vi "Listen.vi"(7 "Listen Address (0=All)":u32 format="%08x", 8 "error in (no error)":errorcluster, 10 "Listen Port (80)":u16=80, 11 "API Queue":refnum<queue>) -> (0 "error out":errorcluster)   [LabVIEW 2023, in "Server.lvclass"]
doc: "Listen on the specified Port. (or on the port stored in the 'Listen Port' VIG)\nAccepts all incoming REST requests, handling them internally if possible. (e.g. static file, control reference endpoint, or event endpoint)\n\nListen Address defaults to all interfaces, either use 'String to IP' to get the network address or 0xCA000001 to only listen on localhost. (The Hex value for 127.0.0.1)"
uses:
  Server.lvclass
  API Message/API Message.lvclass
  Log/Log_Facilities.ctl
  Server.lvclass/Server.ctl
  Log/Log.lvclass
  Request/Request.lvclass
  Response/Response.lvclass
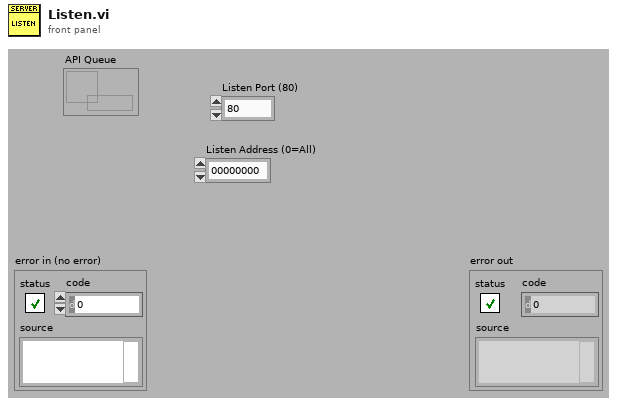
[diagram p1: front panel]
types:
  T1 = typedef "Log.lvclass/Log_Facilities.ctl" = string
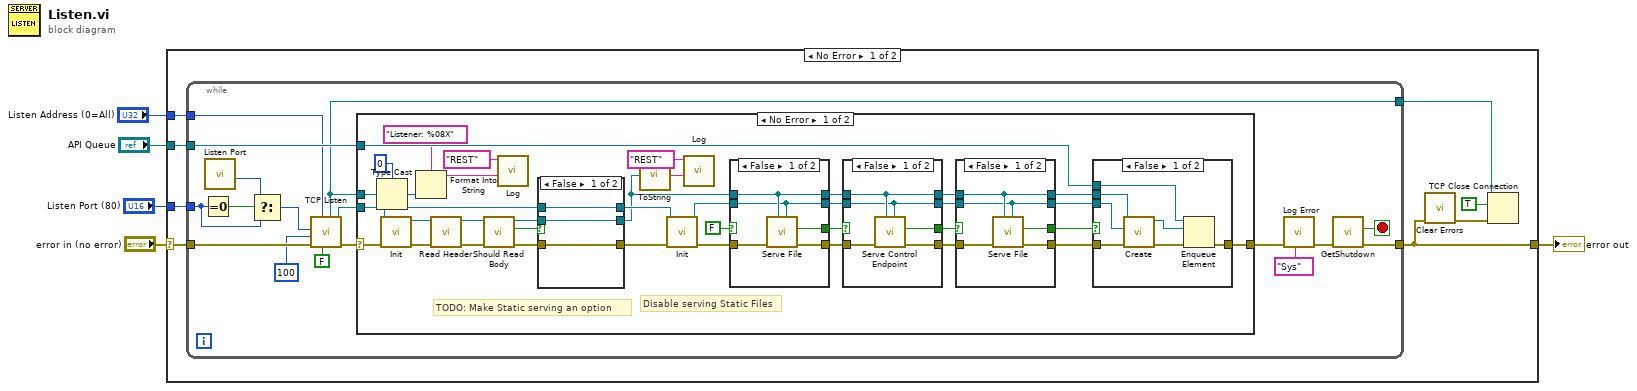
[diagram p0: block diagram]
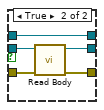
[diagram p6: hidden frame]
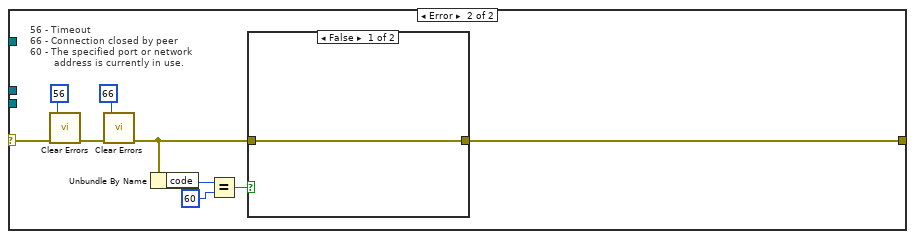
[diagram p7: hidden frame]
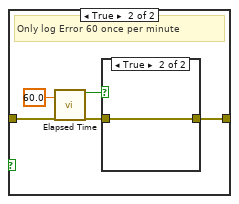
[diagram p8: hidden frame]
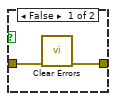
[diagram p9: hidden frame]
diagram:
  n1 = case shown="No Error" "error in (no error)" {
    selector: "error in (no error)" -> [w13 w129]
    tunnel: [w9 w129] -> w4
    tunnel: "API Queue" -> [w12 _]
    tunnel: "Listen Port (80)" -> [w7 _]
    tunnel: "Listen Address (0=All)" -> [w6 _]
    frame No Error {
      n2 = while {
        tunnel: w13 -> [w30]
        tunnel: [w21] -> w9
        tunnel: w12 -> [w23]
        tunnel: [w14] -> w11
        tunnel: w7 -> [w17]
        tunnel: w6 -> [w15]
        stop <- w20 stop-if-true
        n3 = Equal To 0?(x=w17) -> (x = 0?=w19:bool)
        n4 = call "Listen Port.vi"() -> ("Port out"=w18:u16)  [unwired: 11 in]
        n5 = Select(t=w18, s=w19, f=w17) -> (s? t:f=w16:u16)
        n6 = call <vilib>:"TCP Listen.vi"("resolve remote address (T)"=FALSE, "net address"=w15, "error in (no error)"=w30, "timeout ms (wait forever: -1)"=100 ("port"), "port"=w16) -> ("error out"=w27:errorcluster, "connection ID"=w25:refnum<k5>, "listener ID"=w14:refnum<k5>)  [unwired: 2 in, 2 out]
        n7 = case shown="No Error" w27 {
          selector: w27 -> [w67 w117]
          tunnel: w25 -> [w36 _]
          tunnel: [w54 w111] -> w26
          tunnel: w23 -> [w51 _]
          tunnel: w14 -> [w32 _]
          frame No Error {
            # "TODO: Make Static serving an option"
            # "Disable serving Static Files"
            n8 = Type Cast(type=u32 0, x=w32) -> (*(type *) &x=w34:u32)
            n9 = call "Init.vi"("error in (no error)"=w67, "Socket"=w36) -> ("error out"=w60:errorcluster, "Request out"=w62:refnum<class "Request.lvclass">)  [unwired: 8 in]
            n10 = Format Into String(format string="Listener: %08X", w34) -> (resulting string=w35:string)  [unwired: 2 in, 1 out]
            n11 = call "Read Header.vi"("error in (no error)"=w60, "Request in"=w62) -> ("error out"=w59:errorcluster, "Request out"=w61:refnum<class "Request.lvclass">)  [unwired: 8 in]
            n12 = call "Should Read Body.vi"("error in (no error)"=w59, "Request in"=w61) -> ("error out"=w66:errorcluster, "Read Body?"=w64:bool, "Request out"=w65:refnum<class "Request.lvclass">)  [unwired: 7 in]
            n13 = call "Log.vi"("Message"=w35, "Facility"=T1 "REST") -> ()  [unwired: 9 in, 1 out]
            n14 = case shown="False" w64 {
              tunnel: w66 -> [w104 w110]
              tunnel: [w104 w109] -> w58
              tunnel: w65 -> [w105 w108]
              tunnel: [w105 w107] -> w53
              tunnel: w36 -> [w103 w106]
              tunnel: [w103 w106] -> w63
              frame False {
              }
              frame True {
                n15 = call "Read Body.vi"("error in (no error)"=w110, "Request in"=w108) -> ("error out"=w109:errorcluster, "Request out"=w107:refnum<class "Request.lvclass">)  [unwired: 8 in]
              }
            }
            n16 = call "ToString.vi"("Request"=w53) -> ("String"=w57:string)
            n17 = call "Init.vi"("error in (no error)"=w58, "Socket"=w63) -> ("error out"=w56:errorcluster, "Response out"=w52:refnum<class "Response.lvclass">)  [unwired: 8 in]
            n18 = call "Log.vi"("Message"=w57, "Facility"=T1 "REST") -> ()  [unwired: 9 in, 1 out]
            n19 = case shown="False" FALSE {
              selector: FALSE -> [_ w101]
              tunnel: [w98 w102] -> w46
              tunnel: w53 -> [w95 w100]
              tunnel: w52 -> [w94 w99]
              tunnel: w56 -> [w97 w102]
              tunnel: [w96 w101] -> w47
              tunnel: [w95 w100] -> w49
              tunnel: [w94 w99] -> w48
              frame False {
                n20 = call "Serve File.vi"("Response"=w94, "Request"=w95, "error in (no error)"=w97) -> ("error out"=w98:errorcluster, "Handled?"=w96:bool)  [unwired: 7 in]
              }
              frame True {
              }
            }
            n21 = case shown="False" w47 {
              selector: w47 -> [_ w84]
              tunnel: [w80 w85] -> w41
              tunnel: w49 -> [w79 w83]
              tunnel: w48 -> [w78 w82]
              tunnel: w46 -> [w81 w85]
              tunnel: [w77 w84] -> w42
              tunnel: [w79 w83] -> w44
              tunnel: [w78 w82] -> w43
              frame False {
                n22 = call "Serve Control Endpoint.vi"("Response"=w78, "Request"=w79, "error in (no error)"=w81) -> ("error out"=w80:errorcluster, "Handled?"=w77:bool)  [unwired: 7 in]
              }
              frame True {
              }
            }
            n23 = case shown="False" w42 {
              selector: w42 -> [_ w75]
              tunnel: [w72 w76] -> w40
              tunnel: w44 -> [w69 w74]
              tunnel: w43 -> [w68 w73]
              tunnel: w41 -> [w71 w76]
              tunnel: [w70 w75] -> w45
              tunnel: [w69 w74] -> w38
              tunnel: [w68 w73] -> w39
              frame False {
                n24 = call "Serve File.vi"("Response"=w68, "Request"=w69, "error in (no error)"=w71) -> ("error out"=w72:errorcluster, "Handled?"=w70:bool)  [unwired: 7 in]
              }
              frame True {
              }
            }
            n25 = case shown="False" w45 {
              tunnel: [w88 w93] -> w54
              tunnel: w38 -> [w92 _]
              tunnel: w39 -> [w91 _]
              tunnel: w40 -> [w87 w93]
              tunnel: w51 -> [w90 _]
              frame False {
                n26 = call "Create.vi"("error in (no error)"=w87, "Response"=w91, "Request"=w92) -> ("error out"=w86:errorcluster, "API Message out"=w89:refnum<class "API Message.lvclass">)  [unwired: 7 in]
                n27 = Enqueue Element(queue=w90, element=w89, error in (no error)=w86) -> (error out=w88:errorcluster)  [unwired: 1 in, 2 out]
              }
              frame True {
              }
            }
          }
          frame Error {
            # "56 - Timeout\n66 - Connection closed by peer\n60 - The specified port or network \n        address is currently in use."
            n28 = call <vilib>:"Clear Errors.vi"("error in (no error)"=w117, "specific error code to clear (0: all)"=56) -> ("error out"=w116:errorcluster)  [unwired: 4 in, 1 out]
            n29 = call <vilib>:"Clear Errors.vi"("error in (no error)"=w116, "specific error code to clear (0: all)"=66) -> ("error out"=w112:errorcluster)  [unwired: 4 in, 1 out]
            n30 = Unbundle By Name(w112) -> ("code"=w115:i32)
            n31 = Equal?(x=w115, y=60) -> (x = y?=w113:bool)
            n32 = case shown="False" w113 {
              tunnel: w112 -> [w120 w124]
              tunnel: [w120 w121] -> w111
              frame False {
              }
              frame True {
                # "Only log Error 60 once per minute"
                n33 = call "Elapsed Time.vi"("Elapsed Time Target"=60.0, "error in (no error)"=w124) -> ("Time has Elapsed"=w123:bool, "error out"=w122:errorcluster)  [unwired: 12 in, 4 out]
                n34 = case shown="True" w123 {
                  tunnel: w122 -> [w127 w128]
                  tunnel: [w126 w128] -> w121
                  frame False {
                    n35 = call <vilib>:"Clear Errors.vi"("error in (no error)"=w127) -> ("error out"=w126:errorcluster)  [unwired: 5 in, 1 out]
                  }
                  frame True {
                  }
                }
              }
            }
          }
        }
        n36 = call "Log Error.vi"("Facility (default)"=T1 "Sys", "error in (no error)"=w26) -> ("error out"=w22:errorcluster)  [unwired: 9 in]
        n37 = call "GetShutdown.vi"("error in (no error)"=w22) -> ("error out"=w21:errorcluster, "Shutdown"=w20:bool)  [unwired: 9 in]
      }
      n38 = call <vilib>:"Clear Errors.vi"("error in (no error)"=w9) -> ("error out"=w8:errorcluster)  [unwired: 5 in, 1 out]
      n39 = TCP Close Connection(connection ID=w11, abort (F)=TRUE, error in (no error)=w8) -> ()  [unwired: 2 out]
    }
    frame Error {
    }
  }
  "error out" <- w4
